vi "Write TDMS.vi"(8 "error in (no error)":errorcluster, 10 "Array":waveform(dbl)[](array[waveform]), 11 "Refnum in":refnum<k34>) -> (0 "error out":errorcluster, 3 "Refnum out":refnum<k34>)   [LabVIEW 2018, in "TDMS Log.lvlib"]
uses:
  TDMS Log.lvlib
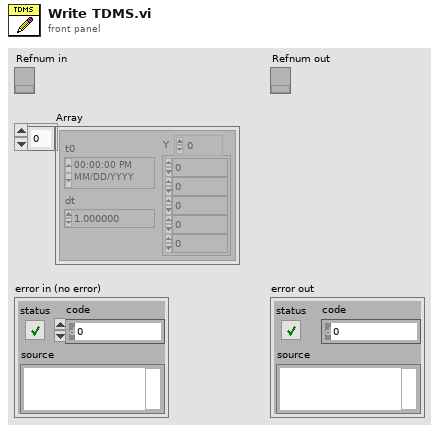
[diagram p1: front panel]
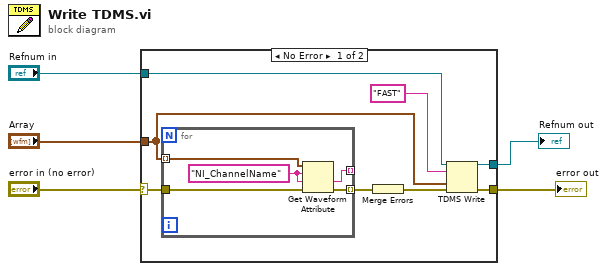
[diagram p0: block diagram]
diagram:
  n1 = case shown="No Error" "error in (no error)" {
    selector: "error in (no error)" -> [w6 w19]
    tunnel: [w12 w19] -> w5
    tunnel: [w11 w20] -> w4
    tunnel: "Refnum in" -> [w10 w20]
    tunnel: "Array" -> [w9 _]
    frame No Error {
      n2 = for {
        tunnel: w9 -> [w18] mode=indexing
        tunnel: [w16] -> _ mode=indexing
        tunnel: [w15] -> w8 mode=indexing
        tunnel: w6 -> [w14]
        w17 = "NI_ChannelName" ("name")
        n3 = Get Waveform Attribute(4:w14, 5:w17, 6:w17, 7:w18) -> (0:w15:errorcluster, 1:w16:string)  [unwired: 2 out]
      }
      n4 = Merge Errors(w8) -> (w7:errorcluster)
      n5 = TDMS Write(0:w10, 5:"FAST" ("group name in (Untitled)"), 9:w9, 11:w7) -> (4:w11:refnum<k34>, 15:w12:errorcluster)  [unwired: 2 in, 2 out]
    }
    frame Error {
    }
  }
  "error out" <- w5
  "Refnum out" <- w4
